vi "显示处理.vi"(9 "项目":i32, 10 "配置文件":string[][](array[string]), 11 "表格":string[][](array[string])) -> (3 "显示":string)   [LabVIEW 2021]
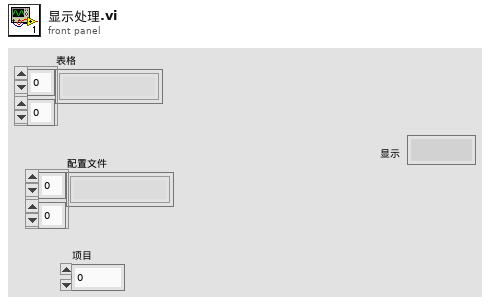
[diagram p1: front panel]
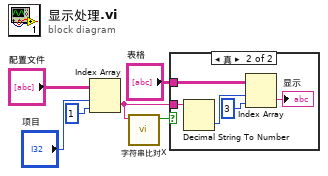
[diagram p0: block diagram]
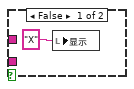
[diagram p2: hidden frame]
diagram:
  n1 = Index Array(array="配置文件", index (row)="项目", index (col)=1 ("禁用的索引 (列)")) -> (element=w4:string)
  n2 = call "字符串比对X.vi"("字符串"=w4) -> ("布尔"=w5:bool)  [unwired: 10 in]
  n3 = case shown="真" w5 {
    tunnel: w4 -> [_ w10]
    tunnel: "表格" -> [_ w9]
    frame False {
      n4 = local write "显示"("X" ("显控6")) -> ()
    }
    frame True {
      n5 = Decimal String To Number(string=w10) -> (number=w11:i32)  [unwired: 2 in, 1 out]
      n6 = Index Array(array=w9, index (row)=w11, index (col)=3 ("禁用的索引 (列)")) -> (element=→"显示":string)
    }
  }
